vi "testTelPacketsSentFromTcpClient.vi"(8 "error in (no error)":errorcluster) -> (0 "error out":errorcluster)   [LabVIEW 2018]
uses:
  src/TcpServer/TcpServer.lvclass/TcpServer.ctl
  src/TcpServerTel/TcpServerTel.lvclass/TcpServerTel.ctl
  <vilib>/addons/_JKI Toolkits/Caraya/classes/Assert/Assert Equal Value_Variant.vi
  src/TcpServerTel/TcpServerTel.lvclass
  <vilib>/addons/_JKI Toolkits/Caraya/classes/Test/Test.lvclass
  src/TcpServer/TcpServer.lvclass
  <vilib>/addons/_JKI Toolkits/Caraya/classes/Assert/Assert.lvclass
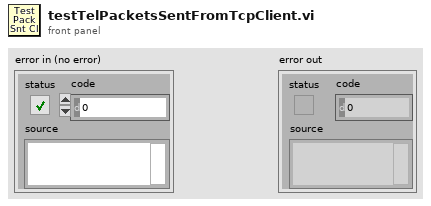
[diagram p1: front panel]
types:
  T1 = cluster{"CmdRead":refnum<user-event>, "EvtRead":refnum<user-event>, "GenRead":refnum<user-event>}
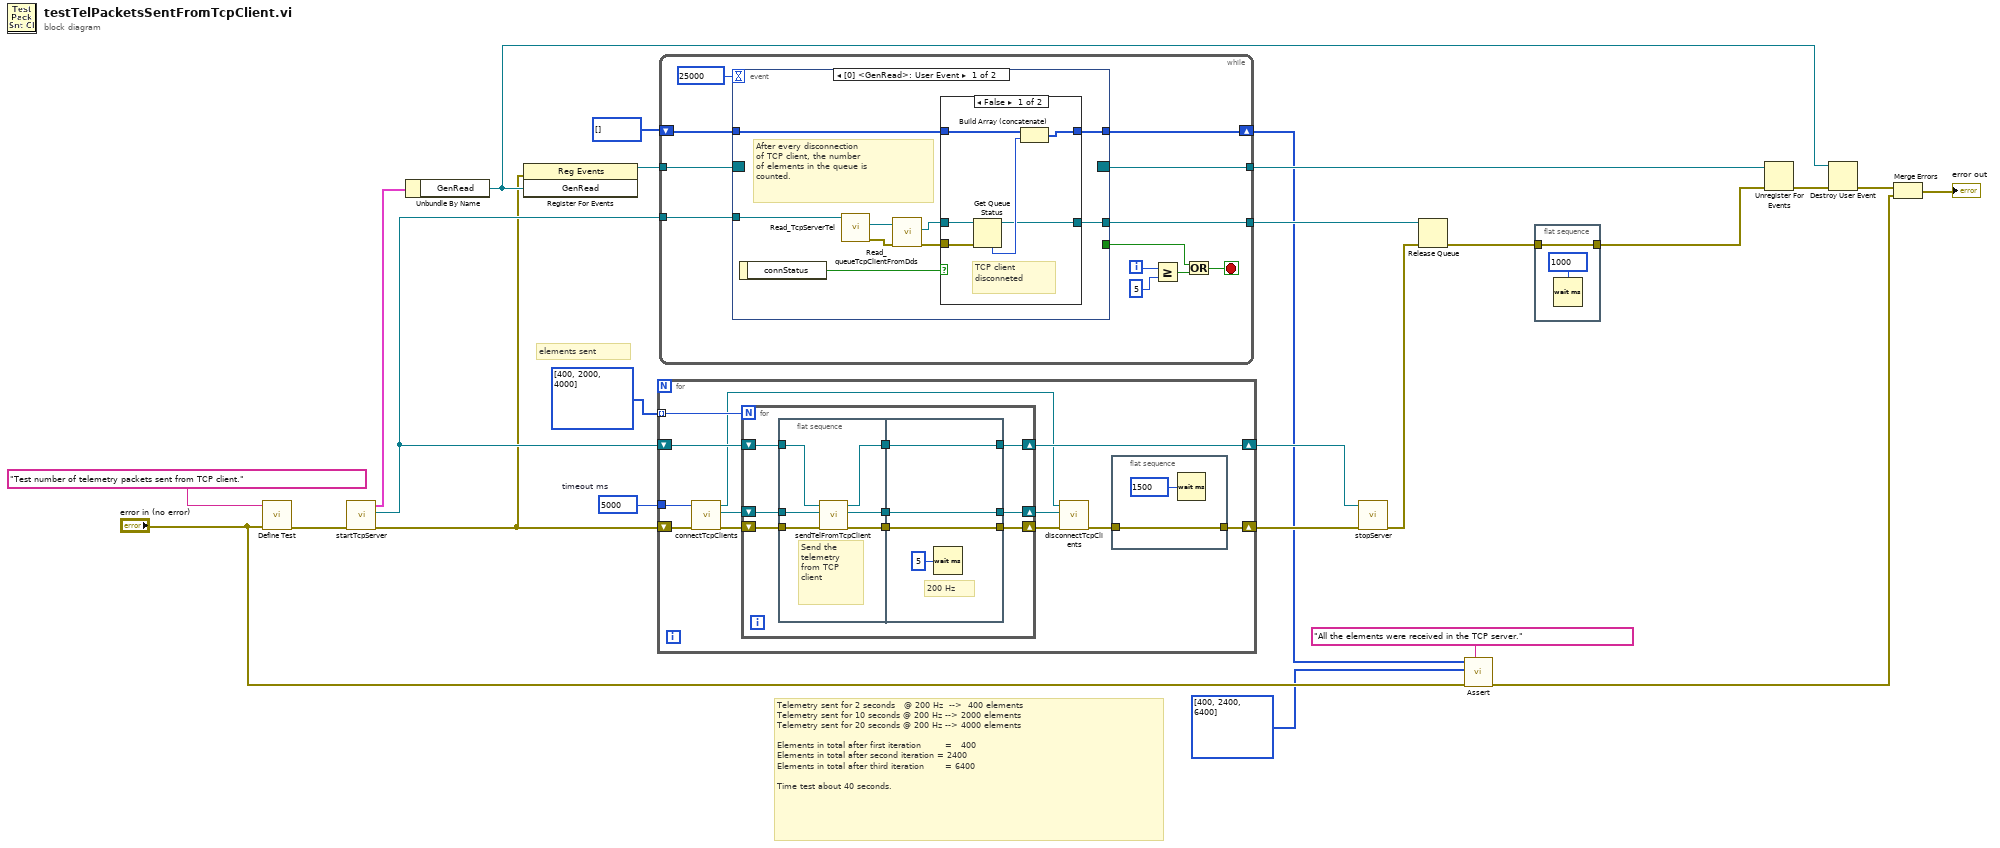
[diagram p0: block diagram]
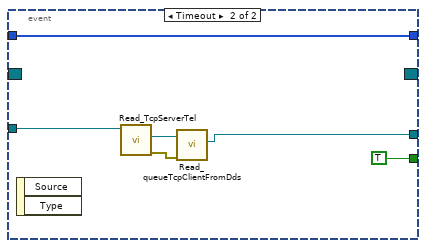
[diagram p3: hidden frame]
diagram:
  w10 = 5000  # timeout ms
  # "elements sent"
  # "Telemetry sent for 2 seconds   @ 200 Hz  -->  400 elements\nTelemetry sent for 10 seconds @ 200 Hz --> 2000 elements\nTelemetry sent for 20 seconds @ 200 Hz --> 4000 elements\n\nElements in total after first iteration        =   400\nElements in total after second iteration = 2400\nElements in total after third iteration       = 6400\n\nTime test about 40 seconds."
  n1 = call <vilib>:"Define Test.vi"("error in (no error)"="error in (no error)", "Label (VI Title)"="Test number of telemetry packets sent from TCP client.") -> ("error out"=w24:errorcluster)  [unwired: 9 in]
  n2 = call "startTcpServer.vi"("error in (no error)"=w24) -> ("error out"=w9:errorcluster, "TcpServer out"=w16:refnum<class "TcpServer.lvclass">, "UserEvents"=w18:T1)  [unwired: 8 in]
  n3 = Unbundle By Name(w18) -> ("GenRead"=w14:refnum<user-event>)
  n4 = register-events(error in=w9, w14) -> (reference out=w17:refnum<event-registration>)  [unwired: 1 in, 1 out]
  n5 = for {
    shift-right: [w27] -> w23
    shift-left: w9 -> [w37]
    shift-right: [w31] -> w21
    shift-left: w16 -> [w36]
    tunnel: i32[] [400, 2000, 4000] -> [w30] mode=indexing
    tunnel: w10 -> [w28]
    n6 = call "connectTcpClients.vi"("error in (no error)"=w37, "timeout ms"=w28) -> ("error out"=w34:errorcluster, "tel connection ID out"=w35:refnum<k5>, "cmd connection ID out"=w29:refnum<k5>)  [unwired: 7 in]
    n7 = for {
      N: w30 -> [_]
      shift-right: [w44] -> w31
      shift-left: w36 -> [w48]
      shift-right: [w43] -> w32
      shift-left: w35 -> [w47]
      shift-right: [w45] -> w33
      shift-left: w34 -> [w46]
      n8 = flat-sequence {
        tunnel: w48 -> [w54]
        tunnel: w47 -> [w53]
        tunnel: w46 -> [w52]
        tunnel: [w51] -> w42
        tunnel: [w50] -> w41
        tunnel: [w49] -> w40
        tunnel: [w56] -> w43
        tunnel: [w57] -> w44
        tunnel: [w58] -> w45
        tunnel: w42 -> [w58]
        tunnel: w41 -> [w57]
        tunnel: w40 -> [w56]
        frame #0 {
          # "Send the\ntelemetry\nfrom TCP\nclient"
          n9 = call "sendTelFromTcpClient.vi"("error in (no error)"=w52, "tel connection ID in"=w53, "TcpServer in"=w54) -> ("error out"=w51:errorcluster, "tel connection ID out"=w49:refnum<k5>, "TcpServer out"=w50:refnum<class "TcpServer.lvclass">)  [unwired: 6 in]
        }
        frame #1 {
          # "200 Hz"
          n10 = Wait (ms)(milliseconds to wait=u32 5) -> ()  [unwired: 1 out]
        }
      }
    }
    n11 = call "disconnectTcpClients.vi"("error in (no error)"=w33, "tel connection ID in"=w32, "cmd connection ID in"=w29) -> ("error out"=w26:errorcluster)  [unwired: 8 in]
    n12 = flat-sequence {
      tunnel: [w38] -> w27
      tunnel: w26 -> [w38]
      frame #0 {
        n13 = Wait (ms)(milliseconds to wait=u32 1500) -> ()  [unwired: 1 out]
      }
    }
  }
  n14 = while {
    tunnel: w17 -> [w70]
    tunnel: w16 -> [w69]
    tunnel: [w68] -> w15
    shift-right: [w66] -> w6
    shift-left: i32[] [] -> [w67]
    tunnel: [w65] -> w8
    i -> [w64]
    stop <- w59 stop-if-true
    n15 = event shown="[0] <GenRead>: User Event" {
      selector: w70 -> [_ _]
      dyn-events: [_ _] -> w68
      timeout: 25000 -> [_ _]
      tunnel: w69 -> [w79 w91]
      tunnel: w67 -> [w73 w89]
      tunnel: [w72 w89] -> w66
      tunnel: [w71 w90] -> w65
      tunnel: [_ TRUE] -> w60
      event User Event {
        # "After every disconnection\nof TCP client, the number \nof elements in the queue is \ncounted."
        n16 = event-data() -> ("connStatus"=w74:bool)  [unwired: 1 in]
        n17 = call "Read_TcpServerTel.vi"("TcpServer in"=w79) -> ("error out"=w76:errorcluster, "TcpServerTel.lvclass"=w75:refnum<class "TcpServerTel.lvclass">)  [unwired: 8 in, 1 out]
        n18 = call "Read_queueTcpClientFromDds.vi"("error in (no error)"=w76, "TcpServerTel in"=w75) -> ("error out"=w78:errorcluster, "queueTcpClientFromDds"=w77:refnum<queue>)  [unwired: 7 in, 1 out]
        n19 = case shown="False" w74 {
          tunnel: w78 -> [w85 _]
          tunnel: w77 -> [w84 w86]
          tunnel: w73 -> [w82 w87]
          tunnel: [w83 w87] -> w72
          tunnel: [w80 w86] -> w71
          frame False {
            # "TCP client\ndisconneted"
            n20 = Get Queue Status(queue=w84, error in (no error)=w85) -> (queue out=w80:refnum<queue>, # elements in queue=w81:i32)  [unwired: 1 in, 6 out]
            n21 = Build Array (concatenate)(w82, w81) -> (w83:i32[])
          }
          frame True {
          }
        }
      }
      event Timeout {
        n22 = event-data() -> ()  [unwired: 1 in, 2 out]
        n23 = call "Read_TcpServerTel.vi"("TcpServer in"=w91) -> ("error out"=w92:errorcluster, "TcpServerTel.lvclass"=w93:refnum<class "TcpServerTel.lvclass">)  [unwired: 8 in, 1 out]
        n24 = call "Read_queueTcpClientFromDds.vi"("error in (no error)"=w92, "TcpServerTel in"=w93) -> ("queueTcpClientFromDds"=w90:refnum<queue>)  [unwired: 7 in, 2 out]
      }
    }
    n25 = Greater Or Equal?(x=w64, y=5) -> (x >= y?=w61:bool)
    n26 = Or(x=w60, y=w61) -> (x .or. y?=w59:bool)
  }
  n27 = call "stopServer.vi"("error in (no error)"=w23, "tcpServer in"=w21) -> ("error out"=w22:errorcluster)  [unwired: 8 in, 1 out]
  n28 = Release Queue(queue=w8, error in (no error)=w22) -> (error out=w4:errorcluster)  [unwired: 1 in, 2 out]
  n29 = call-poly <vilib>:"Assert.vi"("Label"="All the elements were received in the TCP server.", "error in (no error)"="error in (no error)", "Y"=i32[] [400, 2400, 6400], "X"=w6) -> ("error out"=w2:errorcluster)  [unwired: 7 in]
  n30 = flat-sequence {
    tunnel: [w94] -> w5
    tunnel: w4 -> [w94]
    frame #0 {
      n31 = Wait (ms)(milliseconds to wait=u32 1000) -> ()  [unwired: 1 out]
    }
  }
  n32 = Unregister For Events(event registration refnum=w15, error in=w5) -> (error out=w13:errorcluster)
  n33 = Destroy User Event(user event=w14, error in=w13) -> (error out=w3:errorcluster)
  n34 = Merge Errors(w3, w2) -> (→"error out":errorcluster)
